vi "Test_Copy_Image_Greyscale_Mask_Greyscale.vi"(8 "error in (no error)":errorcluster, 11 "Test Case In":refnum<class "Image.lvclass">) -> (0 "error out":errorcluster, 3 "Test Case Out":refnum<class "Image.lvclass">)   [LabVIEW 2020, in "g_ar_toolkit.test.lvlib" / "Image.lvclass"]
uses:
  Image.lvclass
  Image.lvclass/Image.ctl
  g_ar_toolkit.image/g_ar_toolkit.image.lvlib
  g_ar_toolkit.image/Image Size (Fixed).ctl
  g_ar_toolkit.image/CreateEmptyImageGreyscale.vi
  g_ar_toolkit.image/CopyImageMaskGreyscale.vi
  4993e8ee-a06a-463a-9684-69129f64d5ce.vi
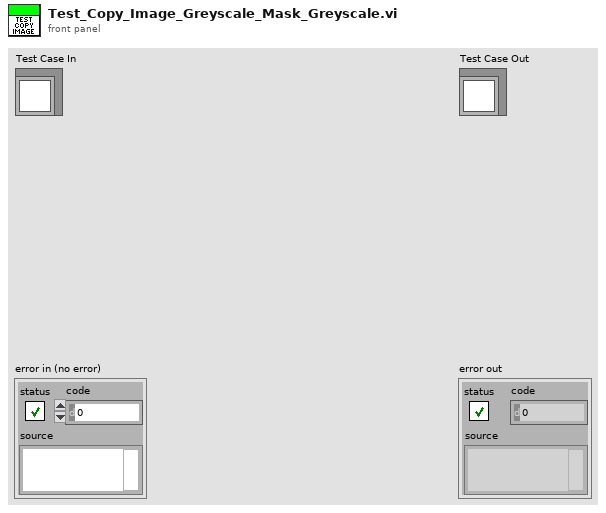
[diagram p1: front panel]
types:
  T1 = typedef "g_ar_toolkit.image.lvlib/Image Size (Fixed).ctl" = cluster{"Width":u16, "Height":u16}
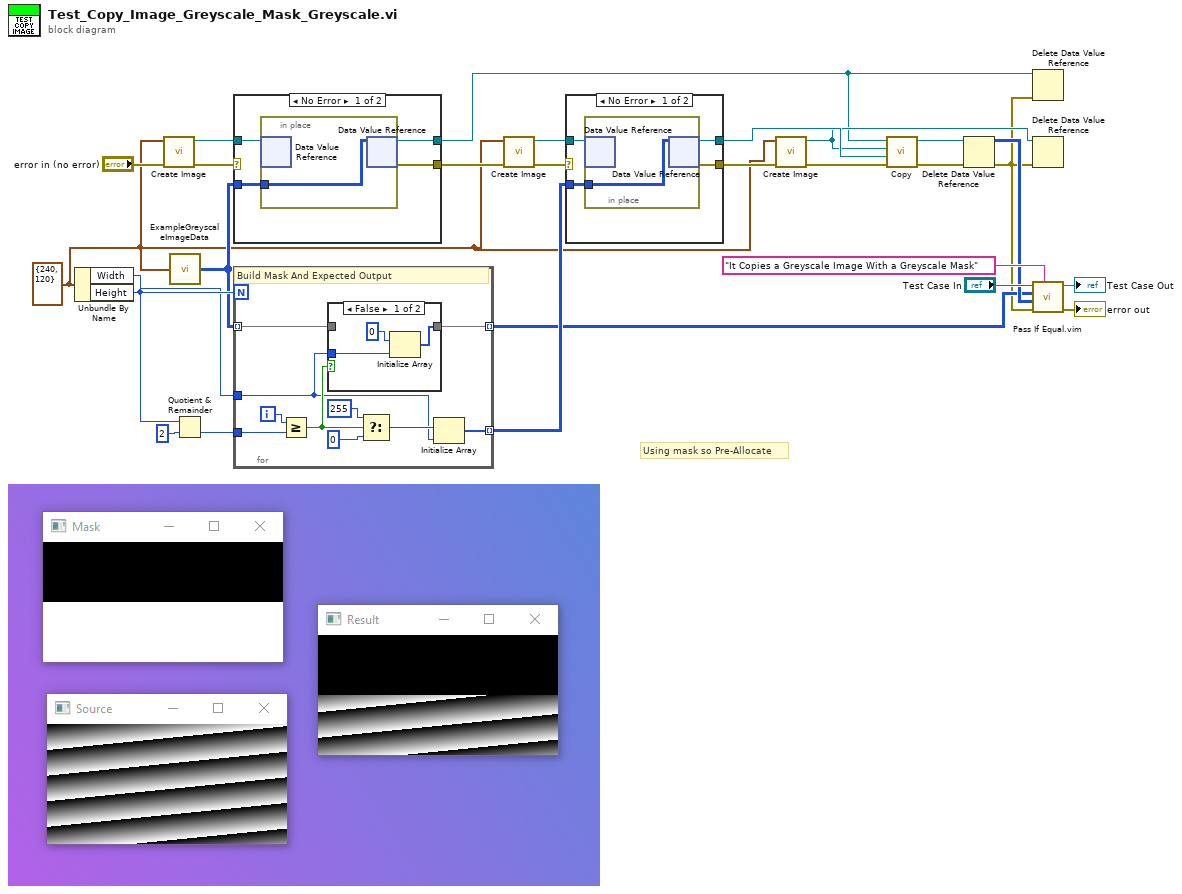
[diagram p0: block diagram]
diagram:
  w1 = T1 {"Width"=240, "Height"=120} ("Preallocated Image Size (Default - 0,0)")
  # "Using mask so Pre-Allocate"
  n1 = Unbundle By Name(w1) -> ("Width"=w12:u16, "Height"=w13:u16)
  n2 = call-poly "Create Image.vi"("error in (no error)"="error in (no error)", "Preallocated Image Size (Default 0,0)"=w1) -> ("error out"=w10:errorcluster, "New Greyscale Image"=w22:refnum<data-value>)  [unwired: 8 in]
  n3 = call "ExampleGreyscaleImageData.vi"("Image Size"=w1) -> ("GreyscaleImage"=w9:u8[][])
  n4 = Quotient & Remainder(x=w13, y=u16 2) -> (floor(x/y)=w11:u16)  [unwired: 1 out]
  n5 = case shown="No Error" w10 {
    selector: w10 -> [_ w34]
    tunnel: w22 -> [w31 w33]
    tunnel: [w30 w34] -> w15
    tunnel: w9 -> [w29 _]
    tunnel: [w28 w33] -> w3
    frame No Error {
      n6 = in-place {
        in-place-border: w29 -> [w32]
        n7 = in-place-dvr #1(w31) -> ()  [unwired: 2 out]
        n8 = in-place-dvr #1(w32) -> (w28:refnum<data-value>, w30:errorcluster)
      }
    }
    frame Error {
    }
  }
  n9 = for {
    N: w13 -> [_]
    tunnel: [w39] -> w19 mode=indexing
    tunnel: w12 -> [w35]
    tunnel: w11 -> [w43]
    tunnel: w9 -> [w38] mode=indexing
    tunnel: [w36] -> w6 mode=indexing
    i -> [w44]
    # "Build Mask And Expected Output"
    n10 = Greater Or Equal?(x=w44, y=w43) -> (x >= y?=w37:bool)
    n11 = case shown="False" w37 {
      tunnel: w38 -> [_ w48]
      tunnel: [w46 w48] -> w36
      tunnel: w35 -> [w47 _]
      frame False {
        n12 = Initialize Array(u8 0, w47) -> (w46:u8[])
      }
      frame True {
      }
    }
    n13 = Select(t=u8 255, s=w37, f=u8 0) -> (s? t:f=w40:u8)
    n14 = Initialize Array(w40, w35) -> (w39:u8[])
  }
  n15 = call-poly "Create Image.vi"("error in (no error)"=w15, "Preallocated Image Size (Default 0,0)"=w1) -> ("error out"=w17:errorcluster, "New Greyscale Image"=w18:refnum<data-value>)  [unwired: 8 in]
  n16 = case shown="No Error" w17 {
    selector: w17 -> [_ w54]
    tunnel: w18 -> [w52 w55]
    tunnel: [w51 w55] -> w8
    tunnel: [w50 w54] -> w16
    tunnel: w19 -> [w49 _]
    frame No Error {
      n17 = in-place {
        in-place-border: w49 -> [w53]
        n18 = in-place-dvr #2(w52) -> ()  [unwired: 2 out]
        n19 = in-place-dvr #2(w53) -> (w51:refnum<data-value>, w50:errorcluster)
      }
    }
    frame Error {
    }
  }
  n20 = call-poly "Create Image.vi"("error in (no error)"=w16, "Preallocated Image Size (Default 0,0)"=w1) -> ("error out"=w21:errorcluster, "New Greyscale Image"=w4:refnum<data-value>)  [unwired: 8 in]
  n21 = call-poly "Copy.vi"("error in (no error)"=w21, "Greyscale Image Mask"=w8, "Greyscale Image Destination"=w4, "Greyscale Image Source"=w3) -> ("error out"=w20:errorcluster, "Greyscale Image Destination (duplicate)"=w5:refnum<data-value>)  [unwired: 6 in]
  n22 = Delete Data Value Reference(data value reference=w5, error in=w20) -> (data value=w7:u8[][], error out=w2:errorcluster)
  n23 = Delete Data Value Reference(data value reference=w3, error in=w2) -> ()  [unwired: 2 out]
  n24 = Delete Data Value Reference(data value reference=w4, error in=w2) -> ()  [unwired: 2 out]
  n25 = call "Pass If Equal.vim"("Description"="It Copies a Greyscale Image With a Greyscale Mask", "error in (no error)"=w2, "Actual"=w7, "Expected"=w6, "LUnit Test Case In"="Test Case In") -> ("error out"=→"error out":errorcluster, "LUnit Test Case Out"=→"Test Case Out":refnum<class "Image.lvclass">)  [unwired: 5 in]
